vi "TagMetadataToImage.vi"(8 "error in (no error)":errorcluster, 10 "Image In":T1, 11 "DemoLasers in":refnum<class "DemoLasers.lvclass">) -> (0 "error out":errorcluster, 2 "Image Out":T1, 3 "DemoLasers out":refnum<class "DemoLasers.lvclass">)   [LabVIEW 2020, in "DemoLasers.lvlib" / "DemoLasers.lvclass"]
uses:
  DemoLasers.lvclass
  <vilib>/vision/Image Controls.llb/IMAQ Image.ctl
  Hardware Abstraction Layer/Component/Laser/Laser/Laser.lvclass
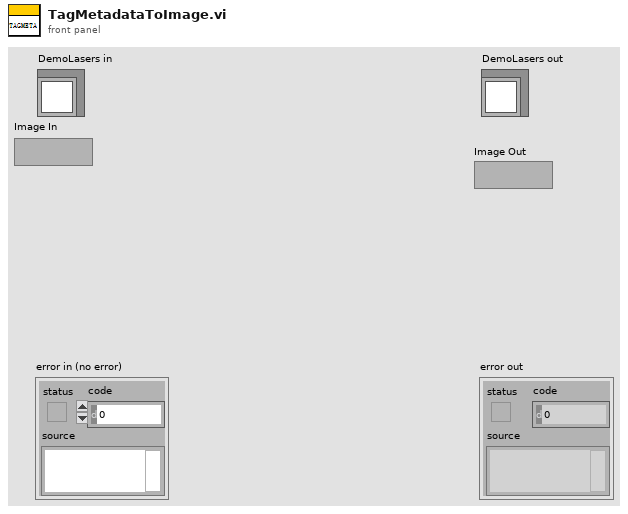
[diagram p1: front panel]
types:
  T1 = typedef "IMAQ Image.ctl" = refnum<image>
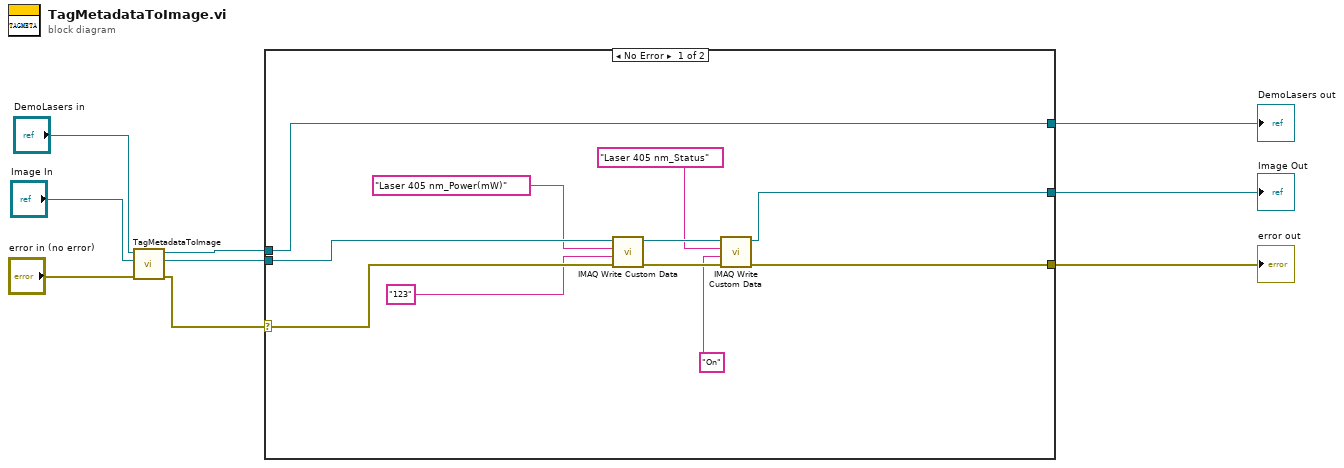
[diagram p0: block diagram]
diagram:
  n1 = call-parent "TagMetadataToImage.vi"("error in (no error)"="error in (no error)", "Image In"="Image In", "Device in"="DemoLasers in") -> ("error out"=w1:errorcluster, "Image Out"=w6:T1, "Device out"=w3:refnum<class "DemoLasers.lvclass">)  [unwired: 6 in]
  n2 = case shown="No Error" w1 {
    selector: w1 -> [w19 w21]
    tunnel: w6 -> [w17 w22]
    tunnel: [w12 w22] -> w5
    tunnel: [w14 w21] -> w4
    tunnel: w3 -> [w20 w23]
    tunnel: [w20 w23] -> w2
    frame No Error {
      n3 = call "IMAQ Write Custom Data"("error in (no error)"=w19, "Custom Data In"="123", "Key"="Laser 405 nm_Power(mW)", "Image"=w17) -> ("error out"=w18:errorcluster, "Image Out"=w13:T1)  [unwired: 6 in]
      n4 = call "IMAQ Write Custom Data"("error in (no error)"=w18, "Custom Data In"="On", "Key"="Laser 405 nm_Status", "Image"=w13) -> ("error out"=w14:errorcluster, "Image Out"=w12:T1)  [unwired: 6 in]
    }
    frame Error {
    }
  }
  "error out" <- w4
  "DemoLasers out" <- w2
  "Image Out" <- w5
